vi "cfgVSI_packet_encoder.vi"(11 "Control settings":T1={"FSM status"=enum."Stopped", "Ctrl bypass"=FALSE, "PID Control"={"Ref_val"=200.0, "Kp"=0.0, "Ti"=0.0, "Td"=0.0, "Out_min"=0.0, "Out_max"=0.0}, "3rd Harmonic"=FALSE, "Output enable"=FALSE, "Phase DBG"=2147} {"Phase DBG" format="%04x"}) -> (3 "concatenated string":string)   [LabVIEW 2015, in "Hardware.lvlib"]
uses:
  Hardware.lvlib
  Settings/VSI Control settings.ctl
  Settings/PID Compensator.ctl
  Settings/Settings.lvlib
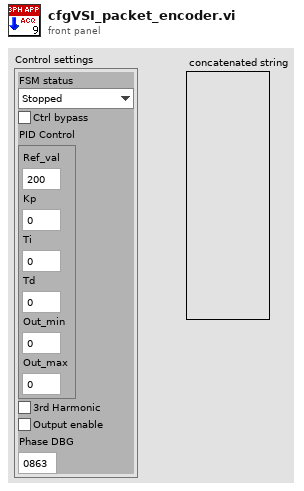
[diagram p1: front panel]
types:
  T1 = typedef "Settings.lvlib/VSI Control settings.ctl" = cluster{"FSM status":enum8{"Stopped", "Running"}, "Ctrl bypass":bool, "PID Control":T2, "3rd Harmonic":bool, "Output enable":bool, "Phase DBG":u32}
  T2 = typedef "Settings.lvlib/PID Compensator.ctl" = cluster{"Ref_val":sgl, "Kp":sgl, "Ti":sgl, "Td":sgl, "Out_min":sgl, "Out_max":sgl}
  T3 = enum16{"big-endian, network order", "native, host order", "little-endian"}
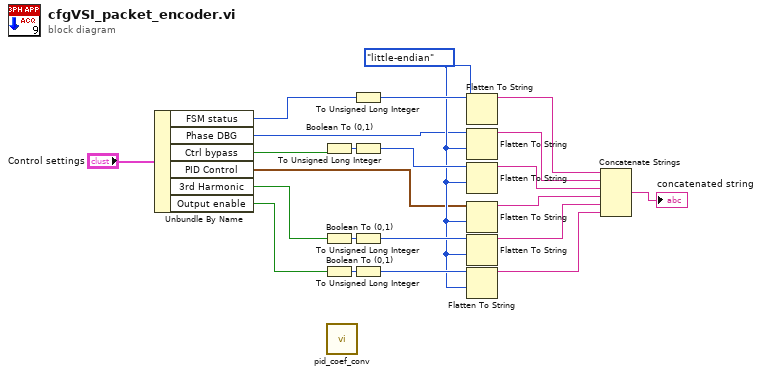
[diagram p0: block diagram]
diagram:
  w4 = T3."little-endian" ("byte order (0:big-endian, network order)")
  n1 = Unbundle By Name("Control settings") -> ("FSM status"=w21:enum8{"Stopped", "Running"}, "Phase DBG"=w2:u32, "Ctrl bypass"=w7:bool, "PID Control"=w1:T2, "3rd Harmonic"=w11:bool, "Output enable"=w12:bool)
  n2 = Boolean To (0,1)(Boolean=w7) -> (0, 1=w6:i16)
  n3 = Boolean To (0,1)(Boolean=w11) -> (0, 1=w9:i16)
  n4 = Boolean To (0,1)(Boolean=w12) -> (0, 1=w8:i16)
  n5 = call "pid_coef_conv.vi"() -> ()  [unwired: 11 in, 1 out]
  n6 = To Unsigned Long Integer(number=w21) -> (unsigned 32bit integer=w19:u32)
  n7 = To Unsigned Long Integer(number=w6) -> (unsigned 32bit integer=w5:u32)
  n8 = To Unsigned Long Integer(number=w9) -> (unsigned 32bit integer=w10:u32)
  n9 = To Unsigned Long Integer(number=w8) -> (unsigned 32bit integer=w13:u32)
  n10 = Flatten To String(anything=w19, byte order (0:big-endian, network order)=w4) -> (data string=w20:string)  [unwired: 2 in, 2 out]
  n11 = Flatten To String(anything=w2, byte order (0:big-endian, network order)=w4) -> (data string=w17:string)  [unwired: 2 in, 2 out]
  n12 = Flatten To String(anything=w5, byte order (0:big-endian, network order)=w4) -> (data string=w3:string)  [unwired: 2 in, 2 out]
  n13 = Flatten To String(anything=w1, byte order (0:big-endian, network order)=w4) -> (data string=w16:string)  [unwired: 2 in, 2 out]
  n14 = Flatten To String(anything=w10, byte order (0:big-endian, network order)=w4) -> (data string=w15:string)  [unwired: 2 in, 2 out]
  n15 = Flatten To String(anything=w13, byte order (0:big-endian, network order)=w4) -> (data string=w14:string)  [unwired: 2 in, 2 out]
  n16 = Concatenate Strings(w20, w17, w3, w16, w15, w14) -> (→"concatenated string":string)
